vi "TestMontage.vi"() -> ()   [LabVIEW 2014]
panel:
  out "Montage":picture
  out "value":dbl[][][](array[numeric])
  in  "Path":path
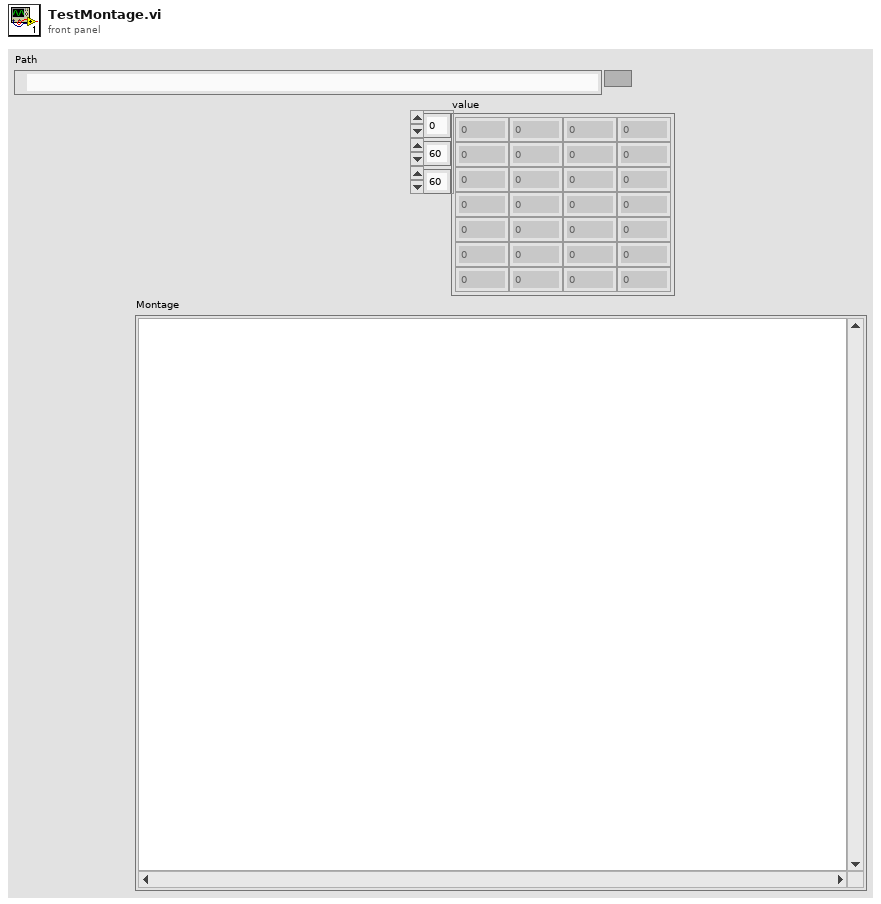
[diagram p1: front panel]
types:
  T1 = enum16{"big-endian, network order", "native, host order", "little-endian"}
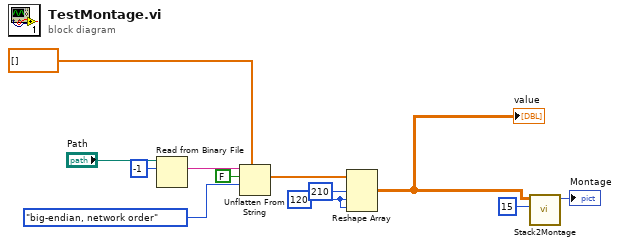
[diagram p0: block diagram]
diagram:
  w4 = 120 ("dimension size")
  n1 = Read from Binary File(10:-1 ("count (1)"), 11:"Path") -> (2:w10:string)  [unwired: 4 in, 3 out]
  n2 = Unflatten From String(type=dbl[] [], binary string=w10, data includes array or string size? (T)=FALSE, byte order (0:big-endian, network order)=T1."big-endian, network order") -> (value=w6:dbl[])  [unwired: 1 in, 2 out]
  n3 = Reshape Array(w6, 210 ("dimension size"), w4, w4) -> (w1:dbl[][][])
  "value" <- w1
  n4 = call "Stack2Montage.vi"("Columns"=15, "StackedAvg"=w1) -> ("Montage"=→"Montage":picture)  [unwired: 8 in, 1 out]
